vi "niDTS BT INSTR RX Configure Trigger.vi"(8 "error in (no error)":errorcluster, 11 "niDTS BT INSTR RX in":refnum<class "niDTS BT INSTR RX.lvclass">) -> (0 "error out":errorcluster, 3 "niDTS BT INSTR RX out":refnum<class "niDTS BT INSTR RX.lvclass">)   [LabVIEW 2015, in "niDTS BT.lvlib" / "niDTS BT INSTR RX.lvclass"]
uses:
  niDTS BT INSTR RX.lvclass
  niDTS BT INSTR RX.lvclass/niDTS BT INSTR RX.ctl
  RiviInstDriver/niRfsgBT/Objects/niRfsgBt.lvclass
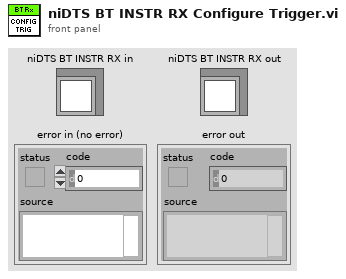
[diagram p1: front panel]
types:
  T1 = typedef "niRfsgBT.lvclass/niRfsgBT INC Handle.ctl" = refnum<data-value>
  T2 = enum16{"IMMediate", "PFI 0", "PFI 1", "RTSI 0", "RTSI 1", "RTSI 2", "RTSI 3", "RTSI 4", "RTSI 5", "RTSI 6", "RTSI 7", "PXI STAR", "Software"}
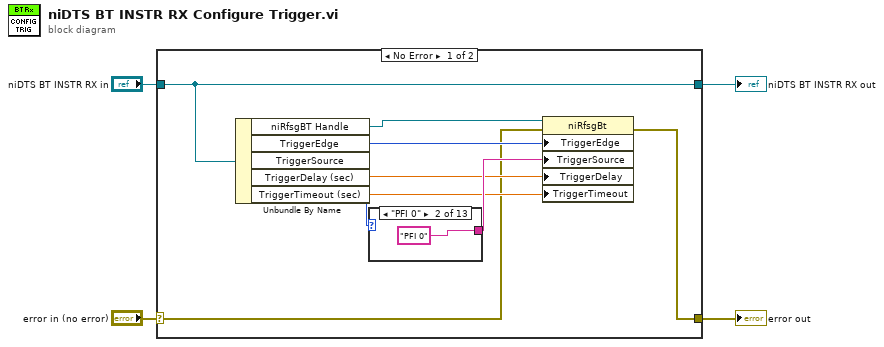
[diagram p0: block diagram]
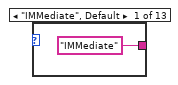
[diagram p2: hidden frame]
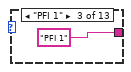
[diagram p3: hidden frame]
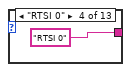
[diagram p4: hidden frame]
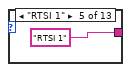
[diagram p5: hidden frame]
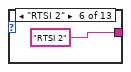
[diagram p6: hidden frame]
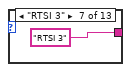
[diagram p7: hidden frame]
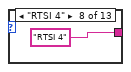
[diagram p8: hidden frame]
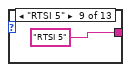
[diagram p9: hidden frame]
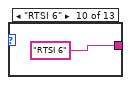
[diagram p10: hidden frame]
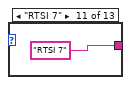
[diagram p11: hidden frame]
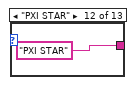
[diagram p12: hidden frame]
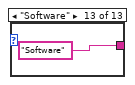
[diagram p13: hidden frame]
diagram:
  n1 = case shown="No Error" "error in (no error)" {
    selector: "error in (no error)" -> [w6 w27]
    tunnel: [w5 w27] -> w3
    tunnel: [w13 w28] -> w1
    tunnel: "niDTS BT INSTR RX in" -> [w13 w28]
    frame No Error {
      n2 = Unbundle By Name(w13) -> ("niRfsgBT Handle"=w12:T1, "TriggerEdge"=w7:enum16{"RISing", "FALLing"}, "TriggerSource"=w10:T2, "TriggerDelay (sec)"=w8:dbl, "TriggerTimeout (sec)"=w9:dbl)
      n3 = case shown="\"PFI 0\"" w10 {
        tunnel: ["IMMediate" ("TRIGger:RFSG:BLUetooth:TriggerSource") "PFI 0" ("TRIGger:RFSG:BLUetooth:TriggerSource") "PFI 1" ("TRIGger:RFSG:BLUetooth:TriggerSource") "RTSI 0" ("TRIGger:RFSG:BLUetooth:TriggerSource") "RTSI 1" ("TRIGger:RFSG:BLUetooth:TriggerSource") "RTSI 2" ("TRIGger:RFSG:BLUetooth:TriggerSource") "RTSI 3" ("TRIGger:RFSG:BLUetooth:TriggerSource") "RTSI 4" ("TRIGger:RFSG:BLUetooth:TriggerSource") "RTSI 5" ("TRIGger:RFSG:BLUetooth:TriggerSource") "RTSI 6" ("TRIGger:RFSG:BLUetooth:TriggerSource") "RTSI 7" ("TRIGger:RFSG:BLUetooth:TriggerSource") "PXI STAR" ("TRIGger:RFSG:BLUetooth:TriggerSource") "Software" ("TRIGger:RFSG:BLUetooth:TriggerSource")] -> w11
        frame "IMMediate", Default {
        }
        frame "PFI 0" {
        }
        frame "PFI 1" {
        }
        frame "RTSI 0" {
        }
        frame "RTSI 1" {
        }
        frame "RTSI 2" {
        }
        frame "RTSI 3" {
        }
        frame "RTSI 4" {
        }
        frame "RTSI 5" {
        }
        frame "RTSI 6" {
        }
        frame "RTSI 7" {
        }
        frame "PXI STAR" {
        }
        frame "Software" {
        }
      }
      n4 = property class="niRfsgBt"(reference=w12, error in=w6, "TriggerEdge"=w7, "TriggerSource"=w11, "TriggerDelay"=w8, "TriggerTimeout"=w9) -> (error out=w5:errorcluster)  [unwired: 1 out]
    }
    frame Error {
    }
  }
  "error out" <- w3
  "niDTS BT INSTR RX out" <- w1
